vi "Main.vi"() -> ()   [LabVIEW 2021]
doc: "Use this template to build a simple state machine design pattern. Each state executes code and determines which state to transition to."
uses:
  Controls/Tic Tac Toe Game Board Boolean Cluster.ctl
  Controls/State.ctl
  Controls/Current System Date & Time.ctl
  Controls/Boolean Text Control States.ctl
panel:
  in  "Tab Control":enum32{"Game", "Back-end Parameters"}(tab)
  out "Current Player's Turn":u16(ring) items=["Currently Player 1 turn", "Currently Player 2 turn"]
  in  "Game Board Cluster":T1
  out "Player 1":string
  out "X Const":string
  out "Player 2":string
  out "O Const":string
  out "Game Win Record":string
  out "Current System Date & Time":T2
  in  "Exit":bool
  out "Stop Clock":bool
  in  "Array - Numeric":dbl[][](array[numeric])
  out "Current State":T3
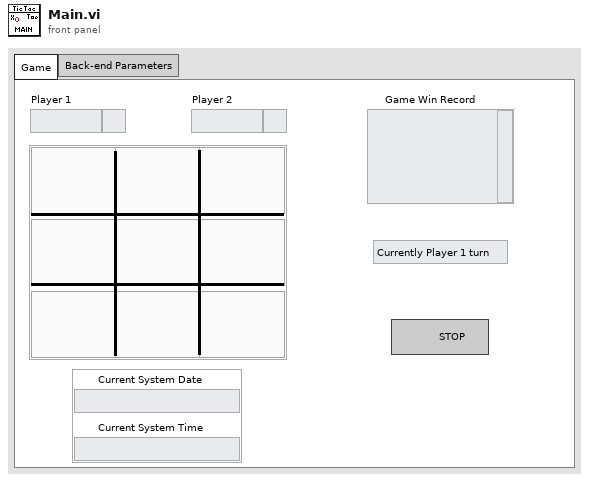
[diagram p1: front panel]
types:
  T1 = typedef "Tic Tac Toe Game Board Boolean Cluster.ctl" = cluster{"Left - Upp":bool, "Left - Mid":bool, "Left - Bot":bool, "Middle - Upp":bool, "Middle - Mid":bool, "Middle - Bot":bool, "Right - Upp":bool, "Right - Mid":bool, "Right - Bot":bool}
  T2 = typedef "Current System Date & Time.ctl" = cluster{"Current System Time":string, "Current System Date":string}
  T3 = typedef "State.ctl" = enum16{"Initialize", "Wait for Event", "Set Left Upp", "Set Left Mid", "Set Left Bot", "Set Middle Upp", "Set Middle Mid", "Set Middle Bot", "Set Right Upp", "Set Right Mid", "Set Right Bot", "Check Game Status", "Exit"}
  T4 = typedef "Boolean Text Control States.ctl" = enum16{"Mark O", "Mark X", "Strike-through O", "Strike-through X"}
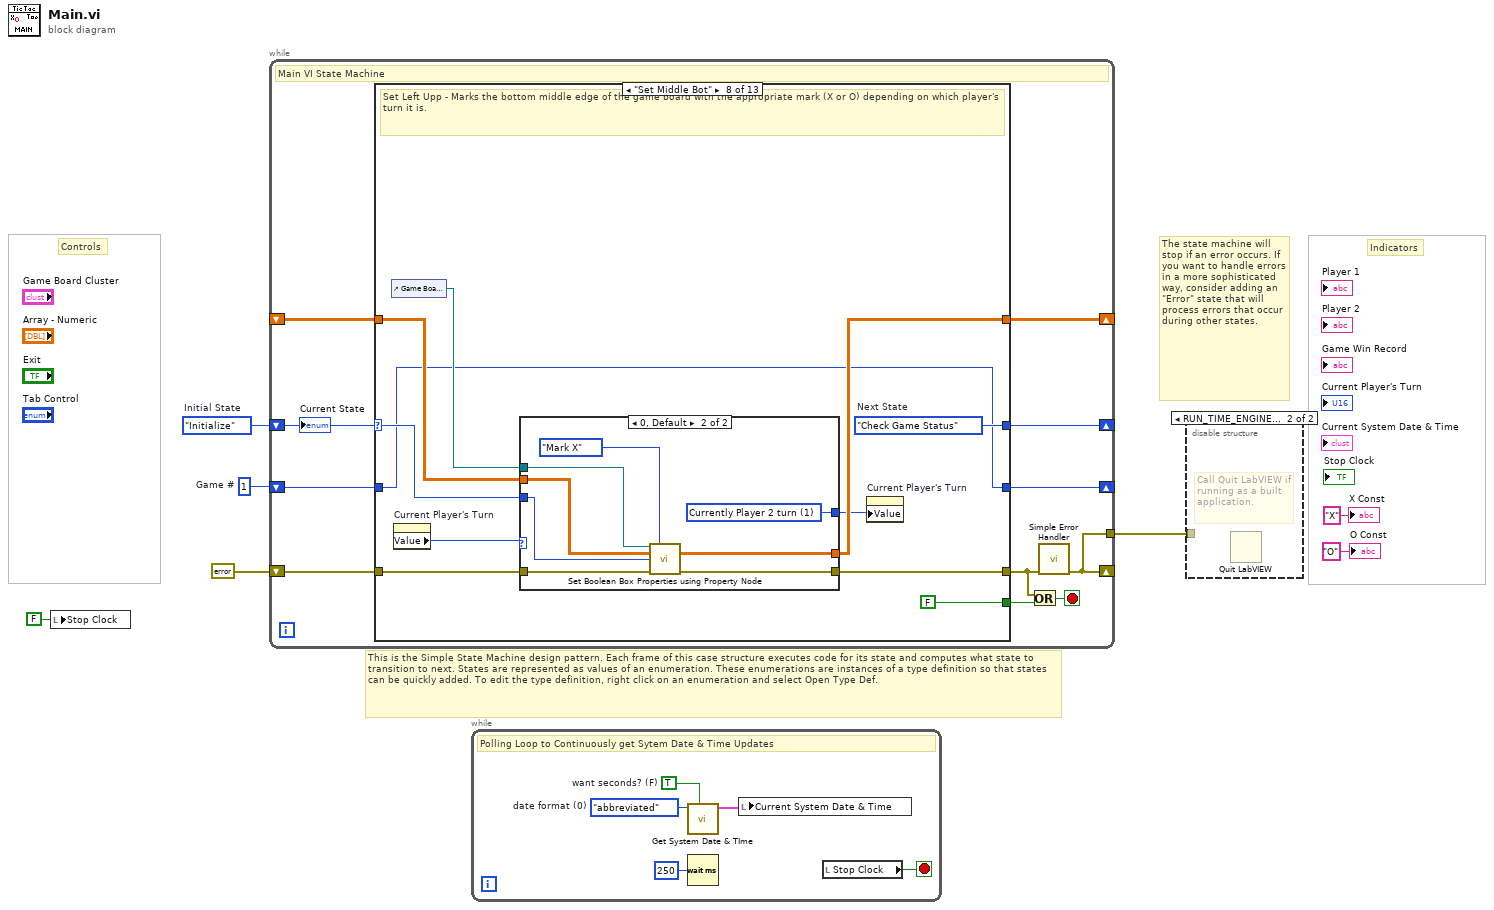
[diagram p0: block diagram]
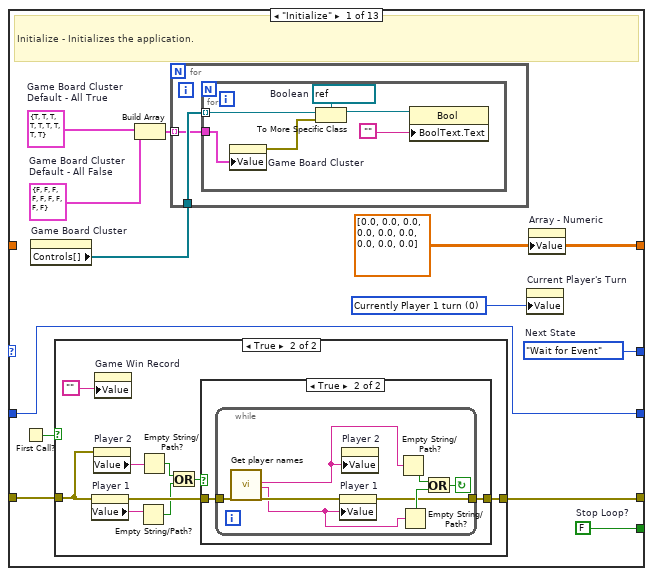
[diagram p3: hidden frame]
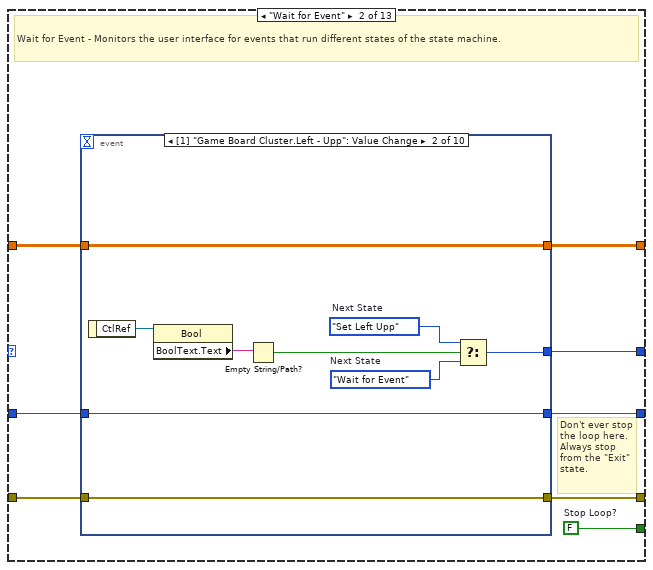
[diagram p6: hidden frame]
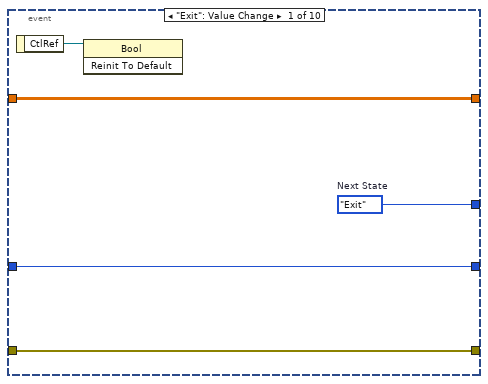
[diagram p7: hidden frame]
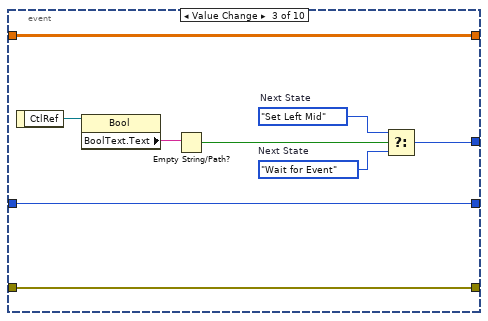
[diagram p8: hidden frame]
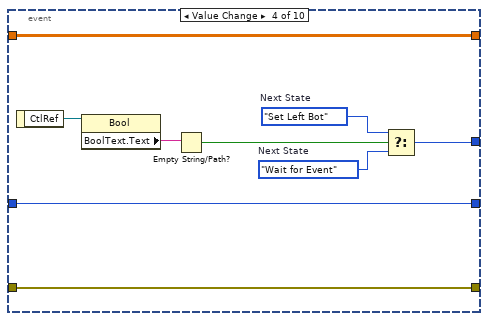
[diagram p9: hidden frame]
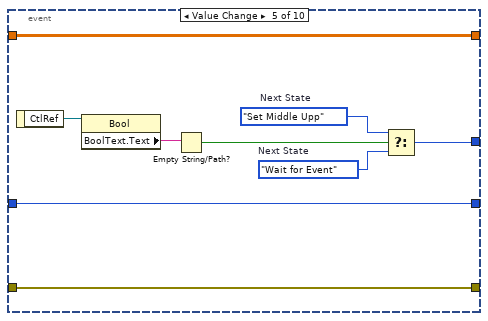
[diagram p10: hidden frame]
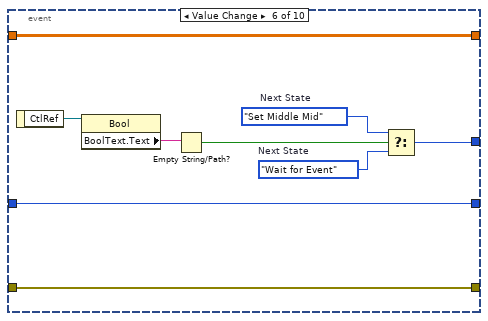
[diagram p11: hidden frame]
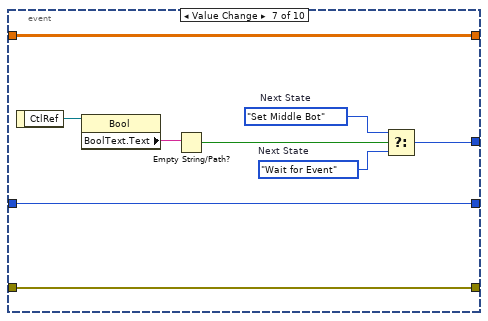
[diagram p12: hidden frame]
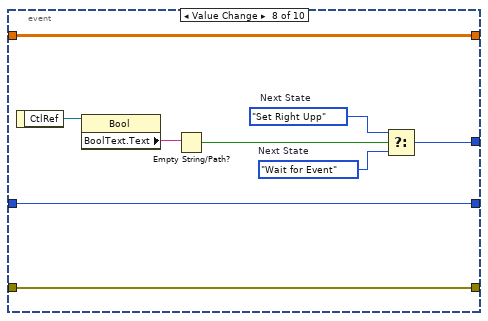
[diagram p13: hidden frame]
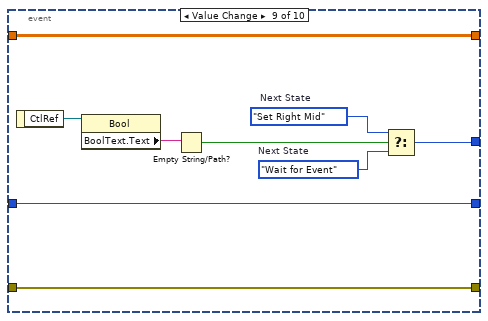
[diagram p14: hidden frame]
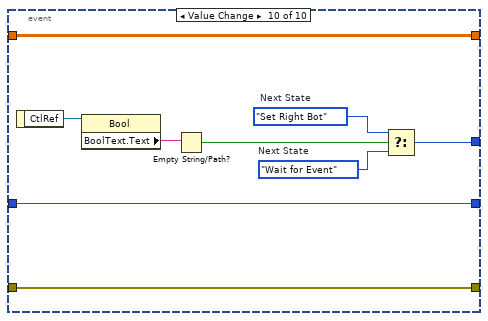
[diagram p15: hidden frame]
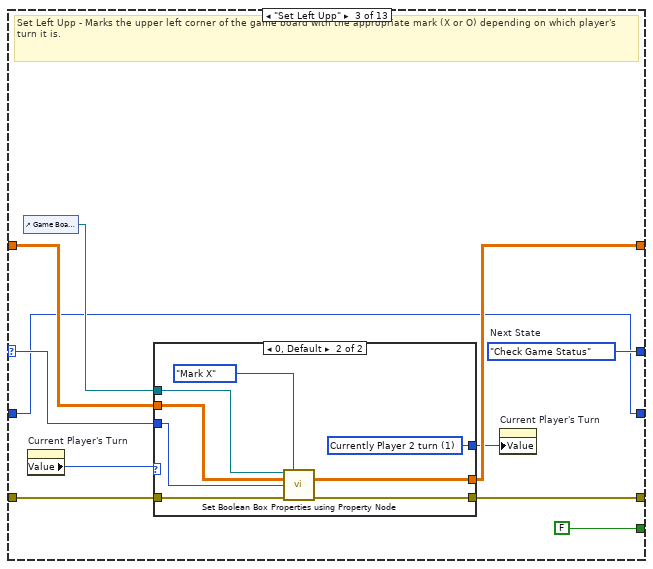
[diagram p16: hidden frame]
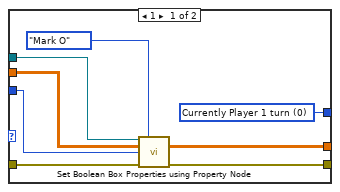
[diagram p17: hidden frame]
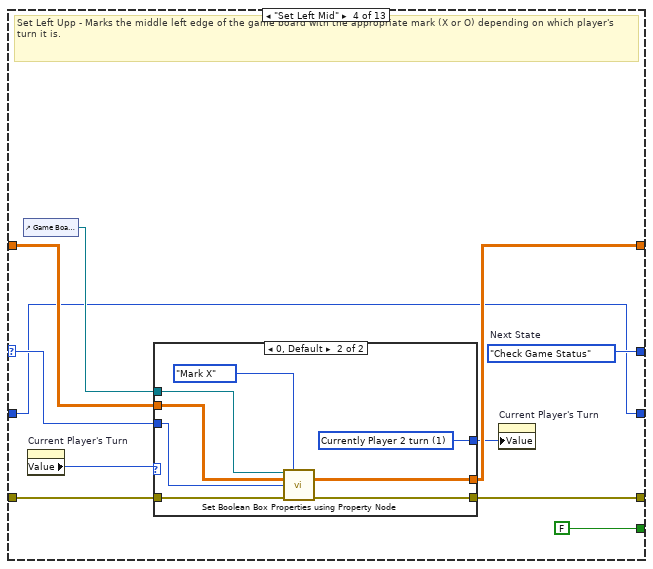
[diagram p18: hidden frame]
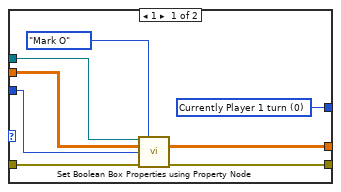
[diagram p19: hidden frame]
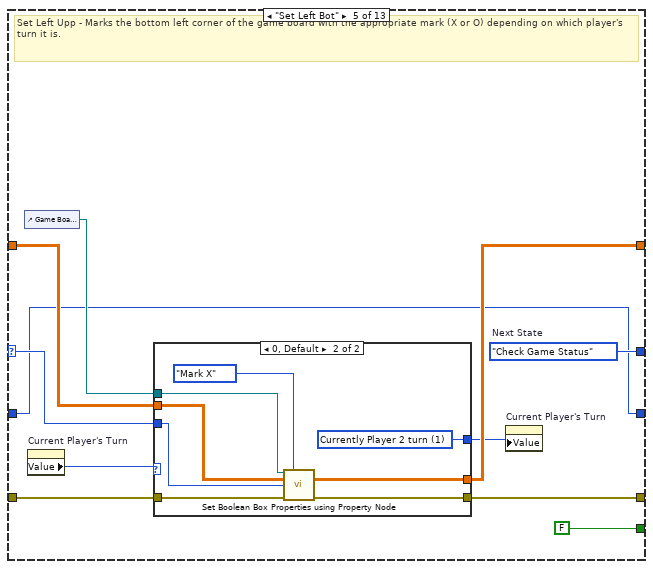
[diagram p20: hidden frame]
diagram:
  w1 = 1  # Game #
  w7 = State."Initialize"  # Initial State
  # "Indicators"
  # "Controls"
  # "The state machine will stop if an error occurs. If you want to handle errors in a more sophisticated way, consider adding an \"Error\" state that will process errors that occur during other states."
  # "This is the Simple State Machine design pattern. Each frame of this case structure executes code for its state and computes what state to transition to next. States are represented as values of an enumeration. These enumerations are instances of a type definition so that states can be quickly added. To edit the type definition, right click on an enumeration and select Open Type Def."
  n1 = local write "Stop Clock"(FALSE ("Stop Clock")) -> ()
  n2 = while {
    shift-right: [w17] -> _
    shift-left: w7 -> [w18]
    shift-right: [w12] -> _
    shift-left: errorcluster {"status"=FALSE, "code"=0, "source"=""} ("error constant") -> [w16]
    shift-right: [w11] -> _
    shift-left: _ -> [w10]
    tunnel: [w12] -> w3
    shift-right: [w8] -> _
    shift-left: w1 -> [w9]
    stop <- w14 stop-if-true
    # "Main VI State Machine"
    n3 = case shown="\"Set Middle Bot\"" w18 {
      selector: w18 -> [_ _ w160 w187 w214 w241 w268 w295 w322 w349 w376 _ _]
      tunnel: [w30 w67 w164 w191 w218 w245 w272 w299 w326 w353 w380 w402 w443] -> w17
      tunnel: [w29 w66 FALSE ("Stop Loop?") FALSE ("Stop Loop?") FALSE ("Stop Loop?") FALSE ("Stop Loop?") FALSE ("Stop Loop?") FALSE ("Stop Loop?") FALSE ("Stop Loop?") FALSE ("Stop Loop?") FALSE ("Stop Loop?") FALSE ("Stop Loop?") w439] -> w15
      tunnel: w16 -> [w28 w65 w162 w189 w216 w243 w270 w297 w324 w351 w378 w407 w442]
      tunnel: [w25 w64 w157 w184 w211 w238 w265 w292 w319 w346 w373 w401 w442] -> w13
      tunnel: [w27 w62 w158 w185 w212 w239 w266 w293 w320 w347 w374 w406 w441] -> w11
      tunnel: w10 -> [_ w63 w159 w186 w213 w240 w267 w294 w321 w348 w375 w406 w441]
      tunnel: w9 -> [w19 w61 w154 w181 w208 w235 w262 w289 w316 w343 w370 w399 w440]
      tunnel: [w19 w60 w154 w181 w208 w235 w262 w289 w316 w343 w370 w398 w440] -> w8
      frame "Initialize" {
        w21 = T1 {"Left - Upp"=FALSE, "Left - Mid"=FALSE, "Left - Bot"=FALSE, "Middle - Upp"=FALSE, "Middle - Mid"=FALSE, "Middle - Bot"=FALSE, "Right - Upp"=FALSE, "Right - Mid"=FALSE, "Right - Bot"=FALSE}  # Game Board Cluster Default - All False
        w24 = u16 0 items=["Currently Player 1 turn", "Currently Player 2 turn"] ("Current Player's Turn")
        w27 = dbl[][] [[0.0, 0.0, 0.0], [0.0, 0.0, 0.0], [0.0, 0.0, 0.0]] ("Array - Numeric")
        w22 = T1 {"Left - Upp"=TRUE, "Left - Mid"=TRUE, "Left - Bot"=TRUE, "Middle - Upp"=TRUE, "Middle - Mid"=TRUE, "Middle - Bot"=TRUE, "Right - Upp"=TRUE, "Right - Mid"=TRUE, "Right - Bot"=TRUE}  # Game Board Cluster Default - All True
        w29 = FALSE  # Stop Loop?
        w30 = State."Wait for Event"  # Next State
        # "Initialize - Initializes the application."
        n4 = First Call?() -> (First Call?: T/F=w26:bool)
        n5 = property on="Game Board Cluster" class="Clust"() -> ("Controls[]"=w23:refnum<vi>[])  [unwired: 2 in, 2 out]
        n6 = case shown="True" w26 {
          tunnel: w28 -> [w39 w48]
          tunnel: [w39 w45] -> w25
          frame False {
          }
          frame True {
            n7 = property on="Player 1" class="Str"(error in=w48) -> (error out=w47:errorcluster, "Value"=w44:string)  [unwired: 1 in, 1 out]
            n8 = property on="Player 2" class="Str"(error in=w48) -> ("Value"=w43:string)  [unwired: 1 in, 2 out]
            n9 = property on="Game Win Record" class="Str"("Value"="") -> ()  [unwired: 2 in, 2 out]
            n10 = Empty String/Path?(string/path=w44) -> (empty?=w41:bool)
            n11 = Empty String/Path?(string/path=w43) -> (empty?=w42:bool)
            n12 = Or(x=w42, y=w41) -> (x .or. y?=w40:bool)
            n13 = case shown="True" w40 {
              tunnel: w47 -> [w49 w51]
              tunnel: [w49 w50] -> w45
              frame False {
              }
              frame True {
                n14 = while {
                  tunnel: w51 -> [w59]
                  tunnel: [w52] -> w50
                  stop <- w53 continue-if-true
                  n15 = call "Get player names"("error in (no error)"=w59) -> ("Player 2:"=w57:string, "Player 1:"=w56:string, "error out"=w58:errorcluster)  [unwired: 15 in, 1 out]
                  n16 = property on="Player 1" class="Str"(error in=w58, "Value"=w56) -> (error out=w52:errorcluster)  [unwired: 1 in, 1 out]
                  n17 = property on="Player 2" class="Str"("Value"=w57) -> ()  [unwired: 2 in, 2 out]
                  n18 = Empty String/Path?(string/path=w57) -> (empty?=w55:bool)
                  n19 = Empty String/Path?(string/path=w56) -> (empty?=w54:bool)
                  n20 = Or(x=w55, y=w54) -> (x .or. y?=w53:bool)
                }
              }
            }
          }
        }
        n21 = Build Array(w22, w21) -> (w20:T1[])
        n22 = for {
          tunnel: w23 -> [w32]
          tunnel: w20 -> [w31] mode=indexing
          n23 = for {
            tunnel: w32 -> [w38] mode=indexing
            tunnel: w31 -> [w34]
            w37 = refnum<vi> refnum  # Boolean
            n24 = property on="Game Board Cluster" class="Clust"("Value"=w34) -> (error out=w35:errorcluster)  [unwired: 2 in, 1 out]
            n25 = To More Specific Class(target class=w37, reference=w38, error in=w35) -> (specific class reference=w36:refnum<vi>)  [unwired: 1 out]
            n26 = property class="Bool"(reference=w36, "BoolText.Text"="") -> ()  [unwired: 1 in, 2 out]
          }
        }
        n27 = property on="Current Player's Turn" class="Ring (strict)"("Value"=w24) -> ()  [unwired: 2 in, 2 out]
        n28 = property on="Array - Numeric" class="Arr (strict)"("Value"=w27) -> ()  [unwired: 2 in, 2 out]
      }
      frame "Wait for Event" {
        w66 = FALSE  # Stop Loop?
        # "Don't ever stop the loop here. Always stop from the \"Exit\" state."
        # "Wait for Event - Monitors the user interface for events that run different states of the state machine."
        n29 = event shown="[1] \"Game Board Cluster.Left - Upp\": Value Change" {
          selector: _ -> [_ _ _ _ _ _ _ _ _ _]
          dyn-events: _ -> [_ _ _ _ _ _ _ _ _ _]
          timeout: _ -> [_ _ _ _ _ _ _ _ _ _]
          tunnel: [w72 w77 w86 w95 w104 w113 w122 w131 w140 w149] -> w67
          tunnel: w65 -> [w71 w81 w90 w99 w108 w117 w126 w135 w144 w153]
          tunnel: [w71 w81 w90 w99 w108 w117 w126 w135 w144 w153] -> w64
          tunnel: w63 -> [w69 w80 w89 w98 w107 w116 w125 w134 w143 w152]
          tunnel: [w69 w80 w89 w98 w107 w116 w125 w134 w143 w152] -> w62
          tunnel: w61 -> [w68 w73 w82 w91 w100 w109 w118 w127 w136 w145]
          tunnel: [w68 w73 w82 w91 w100 w109 w118 w127 w136 w145] -> w60
          event "Exit": Value Change {
            w72 = State."Exit"  # Next State
            n30 = event-data() -> ("CtlRef"=w70:refnum<vi>)  [unwired: 1 in]
            n31 = invoke class="Bool" method="Reinit To Default"(reference=w70) -> ()  [unwired: 2 in, 3 out]
          }
          event Value Change {
            w76 = State."Wait for Event"  # Next State
            w75 = State."Set Left Upp"  # Next State
            n32 = event-data() -> ("CtlRef"=w79:refnum<vi>)  [unwired: 1 in]
            n33 = property class="Bool"(reference=w79) -> ("BoolText.Text"=w78:string)  [unwired: 1 in, 2 out]
            n34 = Empty String/Path?(string/path=w78) -> (empty?=w74:bool)
            n35 = Select(t=w75, s=w74, f=w76) -> (s? t:f=w77:T3)
          }
          event Value Change {
            w85 = State."Wait for Event"  # Next State
            w84 = State."Set Left Mid"  # Next State
            n36 = event-data() -> ("CtlRef"=w88:refnum<vi>)  [unwired: 1 in]
            n37 = property class="Bool"(reference=w88) -> ("BoolText.Text"=w87:string)  [unwired: 1 in, 2 out]
            n38 = Empty String/Path?(string/path=w87) -> (empty?=w83:bool)
            n39 = Select(t=w84, s=w83, f=w85) -> (s? t:f=w86:T3)
          }
          event Value Change {
            w94 = State."Wait for Event"  # Next State
            w93 = State."Set Left Bot"  # Next State
            n40 = event-data() -> ("CtlRef"=w97:refnum<vi>)  [unwired: 1 in]
            n41 = property class="Bool"(reference=w97) -> ("BoolText.Text"=w96:string)  [unwired: 1 in, 2 out]
            n42 = Empty String/Path?(string/path=w96) -> (empty?=w92:bool)
            n43 = Select(t=w93, s=w92, f=w94) -> (s? t:f=w95:T3)
          }
          event Value Change {
            w103 = State."Wait for Event"  # Next State
            w102 = State."Set Middle Upp"  # Next State
            n44 = event-data() -> ("CtlRef"=w106:refnum<vi>)  [unwired: 1 in]
            n45 = property class="Bool"(reference=w106) -> ("BoolText.Text"=w105:string)  [unwired: 1 in, 2 out]
            n46 = Empty String/Path?(string/path=w105) -> (empty?=w101:bool)
            n47 = Select(t=w102, s=w101, f=w103) -> (s? t:f=w104:T3)
          }
          event Value Change {
            w112 = State."Wait for Event"  # Next State
            w111 = State."Set Middle Mid"  # Next State
            n48 = event-data() -> ("CtlRef"=w115:refnum<vi>)  [unwired: 1 in]
            n49 = property class="Bool"(reference=w115) -> ("BoolText.Text"=w114:string)  [unwired: 1 in, 2 out]
            n50 = Empty String/Path?(string/path=w114) -> (empty?=w110:bool)
            n51 = Select(t=w111, s=w110, f=w112) -> (s? t:f=w113:T3)
          }
          event Value Change {
            w121 = State."Wait for Event"  # Next State
            w120 = State."Set Middle Bot"  # Next State
            n52 = event-data() -> ("CtlRef"=w124:refnum<vi>)  [unwired: 1 in]
            n53 = property class="Bool"(reference=w124) -> ("BoolText.Text"=w123:string)  [unwired: 1 in, 2 out]
            n54 = Empty String/Path?(string/path=w123) -> (empty?=w119:bool)
            n55 = Select(t=w120, s=w119, f=w121) -> (s? t:f=w122:T3)
          }
          event Value Change {
            w130 = State."Wait for Event"  # Next State
            w129 = State."Set Right Upp"  # Next State
            n56 = event-data() -> ("CtlRef"=w133:refnum<vi>)  [unwired: 1 in]
            n57 = property class="Bool"(reference=w133) -> ("BoolText.Text"=w132:string)  [unwired: 1 in, 2 out]
            n58 = Empty String/Path?(string/path=w132) -> (empty?=w128:bool)
            n59 = Select(t=w129, s=w128, f=w130) -> (s? t:f=w131:T3)
          }
          event Value Change {
            w139 = State."Wait for Event"  # Next State
            w138 = State."Set Right Mid"  # Next State
            n60 = event-data() -> ("CtlRef"=w142:refnum<vi>)  [unwired: 1 in]
            n61 = property class="Bool"(reference=w142) -> ("BoolText.Text"=w141:string)  [unwired: 1 in, 2 out]
            n62 = Empty String/Path?(string/path=w141) -> (empty?=w137:bool)
            n63 = Select(t=w138, s=w137, f=w139) -> (s? t:f=w140:T3)
          }
          event Value Change {
            w148 = State."Wait for Event"  # Next State
            w147 = State."Set Right Bot"  # Next State
            n64 = event-data() -> ("CtlRef"=w151:refnum<vi>)  [unwired: 1 in]
            n65 = property class="Bool"(reference=w151) -> ("BoolText.Text"=w150:string)  [unwired: 1 in, 2 out]
            n66 = Empty String/Path?(string/path=w150) -> (empty?=w146:bool)
            n67 = Select(t=w147, s=w146, f=w148) -> (s? t:f=w149:T3)
          }
        }
      }
      frame "Set Left Upp" {
        w164 = State."Check Game Status"  # Next State
        # "Set Left Upp - Marks the upper left corner of the game board with the appropriate mark (X or O) depending on which player's turn it is."
        n68 = control-ref of="Game Board Cluster"() -> (w156:refnum<vi>)
        n69 = property on="Current Player's Turn" class="Ring (strict)"() -> ("Value"=w161:u16)  [unwired: 2 in, 2 out]
        n70 = case shown="0, Default" w161 {
          tunnel: w162 -> [w172 w180]
          tunnel: w160 -> [w171 w179]
          tunnel: w159 -> [w170 w178]
          tunnel: [w168 w176] -> w158
          tunnel: [w167 w175] -> w157
          tunnel: w156 -> [w166 w174]
          tunnel: [w165 w173] -> w155
          frame 1 {
            w165 = u16 0 items=["Currently Player 1 turn", "Currently Player 2 turn"] ("Current Player's Turn")
            n71 = call "Set Boolean Box Properties using Property Node.vi"("Game Board Cluster reference"=w166, "Boolean Text Control States"=Boolean_Text_Control_States."Mark O", "Array - In"=w170, "Current State"=w171, "error in (no error)"=w172) -> ("Array - Out"=w168:dbl[][], "error out"=w167:errorcluster)  [unwired: 9 in]
          }
          frame 0, Default {
            w173 = u16 1 items=["Currently Player 1 turn", "Currently Player 2 turn"] ("Current Player's Turn")
            n72 = call "Set Boolean Box Properties using Property Node.vi"("Game Board Cluster reference"=w174, "Boolean Text Control States"=Boolean_Text_Control_States."Mark X", "Array - In"=w178, "Current State"=w179, "error in (no error)"=w180) -> ("Array - Out"=w176:dbl[][], "error out"=w175:errorcluster)  [unwired: 9 in]
          }
        }
        n73 = property on="Current Player's Turn" class="Ring (strict)"("Value"=w155) -> ()  [unwired: 2 in, 2 out]
      }
      frame "Set Left Mid" {
        w191 = State."Check Game Status"  # Next State
        # "Set Left Upp - Marks the middle left edge of the game board with the appropriate mark (X or O) depending on which player's turn it is."
        n74 = control-ref of="Game Board Cluster"() -> (w183:refnum<vi>)
        n75 = property on="Current Player's Turn" class="Ring (strict)"() -> ("Value"=w188:u16)  [unwired: 2 in, 2 out]
        n76 = case shown="0, Default" w188 {
          tunnel: w189 -> [w199 w207]
          tunnel: w187 -> [w198 w206]
          tunnel: w186 -> [w197 w205]
          tunnel: [w195 w203] -> w185
          tunnel: [w194 w202] -> w184
          tunnel: w183 -> [w193 w201]
          tunnel: [w192 w200] -> w182
          frame 1 {
            w192 = u16 0 items=["Currently Player 1 turn", "Currently Player 2 turn"] ("Current Player's Turn")
            n77 = call "Set Boolean Box Properties using Property Node.vi"("Game Board Cluster reference"=w193, "Boolean Text Control States"=Boolean_Text_Control_States."Mark O", "Array - In"=w197, "Current State"=w198, "error in (no error)"=w199) -> ("Array - Out"=w195:dbl[][], "error out"=w194:errorcluster)  [unwired: 9 in]
          }
          frame 0, Default {
            w200 = u16 1 items=["Currently Player 1 turn", "Currently Player 2 turn"] ("Current Player's Turn")
            n78 = call "Set Boolean Box Properties using Property Node.vi"("Game Board Cluster reference"=w201, "Boolean Text Control States"=Boolean_Text_Control_States."Mark X", "Array - In"=w205, "Current State"=w206, "error in (no error)"=w207) -> ("Array - Out"=w203:dbl[][], "error out"=w202:errorcluster)  [unwired: 9 in]
          }
        }
        n79 = property on="Current Player's Turn" class="Ring (strict)"("Value"=w182) -> ()  [unwired: 2 in, 2 out]
      }
      frame "Set Left Bot" {
        w218 = State."Check Game Status"  # Next State
        # "Set Left Upp - Marks the bottom left corner of the game board with the appropriate mark (X or O) depending on which player's turn it is."
        n80 = control-ref of="Game Board Cluster"() -> (w210:refnum<vi>)
        n81 = property on="Current Player's Turn" class="Ring (strict)"() -> ("Value"=w215:u16)  [unwired: 2 in, 2 out]
        n82 = case shown="0, Default" w215 {
          tunnel: w216 -> [w226 w234]
          tunnel: w214 -> [w225 w233]
          tunnel: w213 -> [w224 w232]
          tunnel: [w222 w230] -> w212
          tunnel: [w221 w229] -> w211
          tunnel: w210 -> [w220 w228]
          tunnel: [w219 w227] -> w209
          frame 1 {
            w219 = u16 0 items=["Currently Player 1 turn", "Currently Player 2 turn"] ("Current Player's Turn")
            n83 = call "Set Boolean Box Properties using Property Node.vi"("Game Board Cluster reference"=w220, "Boolean Text Control States"=Boolean_Text_Control_States."Mark O", "Array - In"=w224, "Current State"=w225, "error in (no error)"=w226) -> ("Array - Out"=w222:dbl[][], "error out"=w221:errorcluster)  [unwired: 9 in]
          }
          frame 0, Default {
            w227 = u16 1 items=["Currently Player 1 turn", "Currently Player 2 turn"] ("Current Player's Turn")
            n84 = call "Set Boolean Box Properties using Property Node.vi"("Game Board Cluster reference"=w228, "Boolean Text Control States"=Boolean_Text_Control_States."Mark X", "Array - In"=w232, "Current State"=w233, "error in (no error)"=w234) -> ("Array - Out"=w230:dbl[][], "error out"=w229:errorcluster)  [unwired: 9 in]
          }
        }
        n85 = property on="Current Player's Turn" class="Ring (strict)"("Value"=w209) -> ()  [unwired: 2 in, 2 out]
      }
      frame "Set Middle Upp" {
        w245 = State."Check Game Status"  # Next State
        # "Set Left Upp - Marks the upper middle edge of the game board with the appropriate mark (X or O) depending on which player's turn it is."
        n86 = control-ref of="Game Board Cluster"() -> (w237:refnum<vi>)
        n87 = property on="Current Player's Turn" class="Ring (strict)"() -> ("Value"=w242:u16)  [unwired: 2 in, 2 out]
        n88 = case shown="0, Default" w242 {
          tunnel: w243 -> [w253 w261]
          tunnel: w241 -> [w252 w260]
          tunnel: w240 -> [w251 w259]
          tunnel: [w249 w257] -> w239
          tunnel: [w248 w256] -> w238
          tunnel: w237 -> [w247 w255]
          tunnel: [w246 w254] -> w236
          frame 1 {
            w246 = u16 0 items=["Currently Player 1 turn", "Currently Player 2 turn"] ("Current Player's Turn")
            n89 = call "Set Boolean Box Properties using Property Node.vi"("Game Board Cluster reference"=w247, "Boolean Text Control States"=Boolean_Text_Control_States."Mark O", "Array - In"=w251, "Current State"=w252, "error in (no error)"=w253) -> ("Array - Out"=w249:dbl[][], "error out"=w248:errorcluster)  [unwired: 9 in]
          }
          frame 0, Default {
            w254 = u16 1 items=["Currently Player 1 turn", "Currently Player 2 turn"] ("Current Player's Turn")
            n90 = call "Set Boolean Box Properties using Property Node.vi"("Game Board Cluster reference"=w255, "Boolean Text Control States"=Boolean_Text_Control_States."Mark X", "Array - In"=w259, "Current State"=w260, "error in (no error)"=w261) -> ("Array - Out"=w257:dbl[][], "error out"=w256:errorcluster)  [unwired: 9 in]
          }
        }
        n91 = property on="Current Player's Turn" class="Ring (strict)"("Value"=w236) -> ()  [unwired: 2 in, 2 out]
      }
      frame "Set Middle Mid" {
        w272 = State."Check Game Status"  # Next State
        # "Set Left Upp - Marks the mid middle space of the game board with the appropriate mark (X or O) depending on which player's turn it is."
        n92 = control-ref of="Game Board Cluster"() -> (w264:refnum<vi>)
        n93 = property on="Current Player's Turn" class="Ring (strict)"() -> ("Value"=w269:u16)  [unwired: 2 in, 2 out]
        n94 = case shown="0, Default" w269 {
          tunnel: w270 -> [w280 w288]
          tunnel: w268 -> [w279 w287]
          tunnel: w267 -> [w278 w286]
          tunnel: [w276 w284] -> w266
          tunnel: [w275 w283] -> w265
          tunnel: w264 -> [w274 w282]
          tunnel: [w273 w281] -> w263
          frame 1 {
            w273 = u16 0 items=["Currently Player 1 turn", "Currently Player 2 turn"] ("Current Player's Turn")
            n95 = call "Set Boolean Box Properties using Property Node.vi"("Game Board Cluster reference"=w274, "Boolean Text Control States"=Boolean_Text_Control_States."Mark O", "Array - In"=w278, "Current State"=w279, "error in (no error)"=w280) -> ("Array - Out"=w276:dbl[][], "error out"=w275:errorcluster)  [unwired: 9 in]
          }
          frame 0, Default {
            w281 = u16 1 items=["Currently Player 1 turn", "Currently Player 2 turn"] ("Current Player's Turn")
            n96 = call "Set Boolean Box Properties using Property Node.vi"("Game Board Cluster reference"=w282, "Boolean Text Control States"=Boolean_Text_Control_States."Mark X", "Array - In"=w286, "Current State"=w287, "error in (no error)"=w288) -> ("Array - Out"=w284:dbl[][], "error out"=w283:errorcluster)  [unwired: 9 in]
          }
        }
        n97 = property on="Current Player's Turn" class="Ring (strict)"("Value"=w263) -> ()  [unwired: 2 in, 2 out]
      }
      frame "Set Middle Bot" {
        w299 = State."Check Game Status"  # Next State
        # "Set Left Upp - Marks the bottom middle edge of the game board with the appropriate mark (X or O) depending on which player's turn it is."
        n98 = control-ref of="Game Board Cluster"() -> (w291:refnum<vi>)
        n99 = property on="Current Player's Turn" class="Ring (strict)"() -> ("Value"=w296:u16)  [unwired: 2 in, 2 out]
        n100 = case shown="0, Default" w296 {
          tunnel: w297 -> [w307 w315]
          tunnel: w295 -> [w306 w314]
          tunnel: w294 -> [w305 w313]
          tunnel: [w303 w311] -> w293
          tunnel: [w302 w310] -> w292
          tunnel: w291 -> [w301 w309]
          tunnel: [w300 w308] -> w290
          frame 1 {
            w300 = u16 0 items=["Currently Player 1 turn", "Currently Player 2 turn"] ("Current Player's Turn")
            n101 = call "Set Boolean Box Properties using Property Node.vi"("Game Board Cluster reference"=w301, "Boolean Text Control States"=Boolean_Text_Control_States."Mark O", "Array - In"=w305, "Current State"=w306, "error in (no error)"=w307) -> ("Array - Out"=w303:dbl[][], "error out"=w302:errorcluster)  [unwired: 9 in]
          }
          frame 0, Default {
            w308 = u16 1 items=["Currently Player 1 turn", "Currently Player 2 turn"] ("Current Player's Turn")
            n102 = call "Set Boolean Box Properties using Property Node.vi"("Game Board Cluster reference"=w309, "Boolean Text Control States"=Boolean_Text_Control_States."Mark X", "Array - In"=w313, "Current State"=w314, "error in (no error)"=w315) -> ("Array - Out"=w311:dbl[][], "error out"=w310:errorcluster)  [unwired: 9 in]
          }
        }
        n103 = property on="Current Player's Turn" class="Ring (strict)"("Value"=w290) -> ()  [unwired: 2 in, 2 out]
      }
      frame "Set Right Upp" {
        w326 = State."Check Game Status"  # Next State
        # "Set Left Upp - Marks the upper right corner of the game board with the appropriate mark (X or O) depending on which player's turn it is."
        n104 = control-ref of="Game Board Cluster"() -> (w318:refnum<vi>)
        n105 = property on="Current Player's Turn" class="Ring (strict)"() -> ("Value"=w323:u16)  [unwired: 2 in, 2 out]
        n106 = case shown="0, Default" w323 {
          tunnel: w324 -> [w334 w342]
          tunnel: w322 -> [w333 w341]
          tunnel: w321 -> [w332 w340]
          tunnel: [w330 w338] -> w320
          tunnel: [w329 w337] -> w319
          tunnel: w318 -> [w328 w336]
          tunnel: [w327 w335] -> w317
          frame 1 {
            w327 = u16 0 items=["Currently Player 1 turn", "Currently Player 2 turn"] ("Current Player's Turn")
            n107 = call "Set Boolean Box Properties using Property Node.vi"("Game Board Cluster reference"=w328, "Boolean Text Control States"=Boolean_Text_Control_States."Mark O", "Array - In"=w332, "Current State"=w333, "error in (no error)"=w334) -> ("Array - Out"=w330:dbl[][], "error out"=w329:errorcluster)  [unwired: 9 in]
          }
          frame 0, Default {
            w335 = u16 1 items=["Currently Player 1 turn", "Currently Player 2 turn"] ("Current Player's Turn")
            n108 = call "Set Boolean Box Properties using Property Node.vi"("Game Board Cluster reference"=w336, "Boolean Text Control States"=Boolean_Text_Control_States."Mark X", "Array - In"=w340, "Current State"=w341, "error in (no error)"=w342) -> ("Array - Out"=w338:dbl[][], "error out"=w337:errorcluster)  [unwired: 9 in]
          }
        }
        n109 = property on="Current Player's Turn" class="Ring (strict)"("Value"=w317) -> ()  [unwired: 2 in, 2 out]
      }
      frame "Set Right Mid" {
        w353 = State."Check Game Status"  # Next State
        # "Set Left Upp - Marks the middle right edge of the game board with the appropriate mark (X or O) depending on which player's turn it is."
        n110 = control-ref of="Game Board Cluster"() -> (w345:refnum<vi>)
        n111 = property on="Current Player's Turn" class="Ring (strict)"() -> ("Value"=w350:u16)  [unwired: 2 in, 2 out]
        n112 = case shown="0, Default" w350 {
          tunnel: w351 -> [w361 w369]
          tunnel: w349 -> [w360 w368]
          tunnel: w348 -> [w359 w367]
          tunnel: [w357 w365] -> w347
          tunnel: [w356 w364] -> w346
          tunnel: w345 -> [w355 w363]
          tunnel: [w354 w362] -> w344
          frame 1 {
            w354 = u16 0 items=["Currently Player 1 turn", "Currently Player 2 turn"] ("Current Player's Turn")
            n113 = call "Set Boolean Box Properties using Property Node.vi"("Game Board Cluster reference"=w355, "Boolean Text Control States"=Boolean_Text_Control_States."Mark O", "Array - In"=w359, "Current State"=w360, "error in (no error)"=w361) -> ("Array - Out"=w357:dbl[][], "error out"=w356:errorcluster)  [unwired: 9 in]
          }
          frame 0, Default {
            w362 = u16 1 items=["Currently Player 1 turn", "Currently Player 2 turn"] ("Current Player's Turn")
            n114 = call "Set Boolean Box Properties using Property Node.vi"("Game Board Cluster reference"=w363, "Boolean Text Control States"=Boolean_Text_Control_States."Mark X", "Array - In"=w367, "Current State"=w368, "error in (no error)"=w369) -> ("Array - Out"=w365:dbl[][], "error out"=w364:errorcluster)  [unwired: 9 in]
          }
        }
        n115 = property on="Current Player's Turn" class="Ring (strict)"("Value"=w344) -> ()  [unwired: 2 in, 2 out]
      }
      frame "Set Right Bot" {
        w380 = State."Check Game Status"  # Next State
        # "Set Left Upp - Marks the bottom right corner of the game board with the appropriate mark (X or O) depending on which player's turn it is."
        n116 = control-ref of="Game Board Cluster"() -> (w372:refnum<vi>)
        n117 = property on="Current Player's Turn" class="Ring (strict)"() -> ("Value"=w377:u16)  [unwired: 2 in, 2 out]
        n118 = case shown="0, Default" w377 {
          tunnel: w378 -> [w388 w396]
          tunnel: w376 -> [w387 w395]
          tunnel: w375 -> [w386 w394]
          tunnel: [w384 w392] -> w374
          tunnel: [w383 w391] -> w373
          tunnel: w372 -> [w382 w390]
          tunnel: [w381 w389] -> w371
          frame 1 {
            w381 = u16 0 items=["Currently Player 1 turn", "Currently Player 2 turn"] ("Current Player's Turn")
            n119 = call "Set Boolean Box Properties using Property Node.vi"("Game Board Cluster reference"=w382, "Boolean Text Control States"=Boolean_Text_Control_States."Mark O", "Array - In"=w386, "Current State"=w387, "error in (no error)"=w388) -> ("Array - Out"=w384:dbl[][], "error out"=w383:errorcluster)  [unwired: 9 in]
          }
          frame 0, Default {
            w389 = u16 1 items=["Currently Player 1 turn", "Currently Player 2 turn"] ("Current Player's Turn")
            n120 = call "Set Boolean Box Properties using Property Node.vi"("Game Board Cluster reference"=w390, "Boolean Text Control States"=Boolean_Text_Control_States."Mark X", "Array - In"=w394, "Current State"=w395, "error in (no error)"=w396) -> ("Array - Out"=w392:dbl[][], "error out"=w391:errorcluster)  [unwired: 9 in]
          }
        }
        n121 = property on="Current Player's Turn" class="Ring (strict)"("Value"=w371) -> ()  [unwired: 2 in, 2 out]
      }
      frame "Check Game Status" {
        # "Check Game Status - Checks to see if the game has been won and displays the proper UI information if it has.  If the game has been won then the users can choose to play again or exit.\nIf the game has not been run then it will just resume play."
        n122 = call "Check for Game Winner.vi"("error in"=w407, "Array - Numeric"=w406) -> ("error out"=w405:errorcluster, "Tie Game"=w397:bool, "Player 1 wins"=w403:bool, "Game Won"=w404:bool)  [unwired: 6 in]
        n123 = case shown="False" w404 {
          tunnel: w405 -> [w412 w437]
          tunnel: w403 -> [_ w438]
          tunnel: [w410 w430] -> w402
          tunnel: [w411 w436] -> w401
          tunnel: w399 -> [w409 w428]
          tunnel: [w408 w427] -> w398
          tunnel: w397 -> [w413 _]
          frame False {
            # "This case is executed if the game has been not been won."
            n124 = case shown="True" w413 {
              tunnel: w412 -> [w416 w419]
              tunnel: [w416 w418] -> w411
              tunnel: [w415 w417] -> w410
              tunnel: [w414 w420] -> w408
              tunnel: w409 -> [w414 w421]
              frame False {
                w415 = State."Wait for Event"  # Next State
                # "This case is executed if the game is to resume (no winer yet)."
              }
              frame True {
                # "This case is executed if the game ended in a tie."
                n125 = local read "Game Win Record"() -> (w425:string)
                n126 = call "Tie Game User Prompt and State Transition Out.vi"("error in (no error)"=w419) -> ("error out"=w418:errorcluster, "Next State - Out"=w417:T3)  [unwired: 9 in]
                n127 = Number To Decimal String(number=w421) -> (decimal integer string=w422:string)  [unwired: 1 in]
                n128 = Increment(x=w421) -> (x+1=w420:i32)
                n129 = Concatenate Strings(w425, "\r", "It is a tie for game #" ("string"), w422) -> (w426:string)
                n130 = local write "Game Win Record"(w426) -> ()
              }
            }
          }
          frame True {
            # "This case is executed if the game has been won."
            n131 = call "Won Game User Prompt and State Transition Out.vi"("error in (no error)"=w437, "Player 1 wins"=w438) -> ("error out"=w436:errorcluster, "Next State - Out"=w430:T3, "String - Out"=w429:string)  [unwired: 7 in]
            n132 = local read "Game Win Record"() -> (w433:string)
            n133 = Number To Decimal String(number=w428) -> (decimal integer string=w435:string)  [unwired: 1 in]
            n134 = Increment(x=w428) -> (x+1=w427:i32)
            n135 = Concatenate Strings(w433, "\r", w429, " game #" ("string"), w435) -> (w434:string)
            n136 = local write "Game Win Record"(w434) -> ()
          }
        }
      }
      frame "Exit" {
        w443 = State."Exit"  # (Value Not Used)
        # "The state value is not used here since this is the last iteration of the state machine loop."
        # "Exit - Exits the application."
        n137 = disable-structure shown="Disabled" {
          frame Disabled {
            n138 = flat-sequence {
              tunnel: [w452] -> w450
              tunnel: [w451] -> w449
              tunnel: w450 -> [w454]
              tunnel: [w454] -> w448
              tunnel: w449 -> [w453]
              tunnel: [w453] -> w447
              tunnel: w448 -> [w457]
              tunnel: w447 -> [w458]
              frame #0 {
                n139 = property on="Player 1" class="Str"() -> ("Value"=w452:string)  [unwired: 2 in, 2 out]
                n140 = property on="Player 2" class="Str"() -> ("Value"=w451:string)  [unwired: 2 in, 2 out]
              }
              frame #1 {
                n141 = control-ref of="This VI"() -> (w456:refnum<vi>)
                n142 = invoke class="VI" method="Default Vals.Reinit All"(reference=w456) -> (reference out=w455:refnum<vi>)  [unwired: 2 in, 2 out]
                n143 = Close Reference(reference=w455) -> ()  [unwired: 1 in, 1 out]
              }
              frame #2 {
                n144 = property on="Player 1" class="Str"("Value"=w457) -> ()  [unwired: 2 in, 2 out]
                n145 = property on="Player 2" class="Str"("Value"=w458) -> ()  [unwired: 2 in, 2 out]
              }
            }
          }
          frame Enabled {
          }
        }
        n146 = flat-sequence {
          tunnel: [w446] -> w439
          frame #0 {
            n147 = control-ref of="This VI"() -> (w444:refnum<vi>)
            n148 = invoke class="VI" method="Default Vals.Reinit All"(reference=w444) -> (reference out=w445:refnum<vi>)  [unwired: 2 in, 2 out]
            n149 = Close Reference(reference=w445) -> ()  [unwired: 1 in, 1 out]
          }
          frame #1 {
            w446 = TRUE  # Stop Loop?
            n150 = local write "Stop Clock"(w446) -> ()
          }
        }
      }
    }
    n151 = Or(x=w13, y=w15) -> (x .or. y?=w14:bool)
    n152 = call <vilib>:"Simple Error Handler.vi"("error in (no error)"=w13) -> ("error out"=w12:errorcluster)  [unwired: 4 in, 4 out]
    "Current State" <- w18
  }
  n153 = while {
    stop <- w459 stop-if-true
    w461 = enum16{"short", "long", "abbreviated"}."abbreviated"  # date format (0)
    w462 = TRUE  # want seconds? (F)
    # "Polling Loop to Continuously get Sytem Date & Time Updates"
    n154 = call "Get System Date & TIme.vi"("want seconds? (F)"=w462, "date format (0)"=w461) -> ("Current System Date & Time"=w463:T2)  [unwired: 9 in]
    n155 = Wait (ms)(milliseconds to wait=u32 250) -> ()  [unwired: 1 out]
    n156 = local write "Current System Date & Time"(w463) -> ()
    n157 = local read "Stop Clock"() -> (w459:bool)
  }
  n158 = disable-structure shown="RUN_TIME_ENGINE==True" {
    disable-tunnel: w3 -> [_ _]
    frame condition #0 (active) {
    }
    frame condition #1 {
      # "Call Quit LabVIEW if running as a built application."
      n159 = Quit LabVIEW() -> ()  [unwired: 1 in]
    }
  }
  "X Const" <- "X" ("X Const")
  "O Const" <- "O" ("O Const")
